vi "Initialize Block.vi"(9 "Outputs":refnum<class "Output.lvclass">[](array[class]), 10 "Inputs":refnum<class "Input.lvclass">[](array[class]), 11 "Block Type":refnum<class "Block.lvclass">) -> (3 "Initialized Block":refnum<class "Block.lvclass">)   [LabVIEW 2020, in "Parallel Block.lvlib" / "Manager.lvclass"]
uses:
  Manager.lvclass
  Manager.lvclass/Manager.ctl
  Block/Block.lvclass
  Input/Input.lvclass
  Output/Output.lvclass
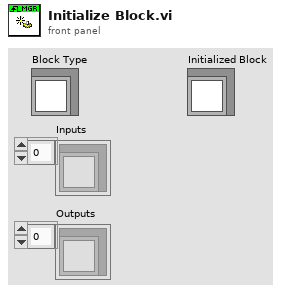
[diagram p1: front panel]
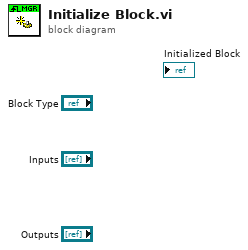
[diagram p0: block diagram]
diagram:
